vi "PID control for simple Suspension System.vi"() -> ()   [LabVIEW 2014]
uses:
  <vilib>/Simulation/Scripting/Companion Diagram/SimConfigNode/SimParams.ctl
  <vilib>/Simulation/Scripting/Companion Diagram/SimConfigNode/_simSolvers.ctl
  <vilib>/Simulation/Implementation/Shared/SIMSCR Execution Mode.ctl
  <vilib>/Simulation/Param Hierarchy/Typedefs/SIMPH Param Control Actions.ctl
  <vilib>/Simulation/Implementation/Shared/SIM limit type.ctl
  <vilib>/Simulation/Implementation/Shared/NILVSim_ParamChanged.vi
  <vilib>/Simulation/Implementation/Shared/NILVSIM_BeginStep.vi
  <vilib>/Simulation/DataSources/Implementation/NILVSim Step.llb/SIM Step (scalar).vi
  <vilib>/Simulation/ContinuousLinear/Implementation/NILVSim Integrator new.llb/SIM Integrator distributor (scalar).vi
  <vilib>/Simulation/SignalDisplay/Implementation/NILVSim Time Waveform.llb/SIM Time Waveform (vector).vi
  <vilib>/Simulation/Utility/Implementation/NILVSim Memory.llb/NILVSim Memory (core).vi
  <vilib>/Simulation/SignalArithmetic/Implementation/NILVSim Gain.llb/SIM Gain (scalar).vi
  <vilib>/Simulation/ContinuousLinear/Implementation/NILVSim Derivative.llb/SIM derivative (scalar).vi
  <vilib>/Simulation/ContinuousLinear/Implementation/NILVSim Integrator new.llb/SIM Integrator collector (scalar).vi
  <vilib>/Simulation/Implementation/Shared/NILVSim_Manager.vi
  <vilib>/Utility/error.llb/Clear Errors.vi
  <vilib>/Simulation/Implementation/Shared/NILVSim_FinalizeModel.vi
  <vilib>/Simulation/Implementation/Shared/SIM Unbundle Sim Info.vi
  <vilib>/Simulation/Implementation/Shared/NILVSim_Initialize.vi
  <vilib>/Simulation/Utility/Implementation/NILVSim Get Time and IsAcceptedStep.vi
  <vilib>/Simulation/Implementation/Shared/SIMSH Read Queue.vi
  <vilib>/Simulation/Implementation/Shared/NILVSim_GetModelError.vi
  <vilib>/Simulation/Implementation/Shared/SIM Bundle Sim Info.vi
  <vilib>/imath/engines/lvmath/Plug In/Control Design/BuiltInFunctions/tf/NIMS_CD_tf(num,den,Ts).vi
  <vilib>/imath/engines/lvmath/Plug In/Control Design/BuiltInFunctions/plus/NIMS_CD_plus(TF,TF).vi
  <vilib>/imath/engines/lvmath/Functions/Error Handling/MergeErrorsWrapper.vi
  <vilib>/imath/engines/lvmath2/RunTimeEngine/NodeEndStatement/NIMS_NodeEndStatement_Output.vi
  <instcachedir>/0/NIMS_NodeEndStatement_Output_53EC0D466D134D7ABD903AC30B43404B.lvgen/NIMS_NodeEndStatement_Output_53EC0D466D134D7ABD903AC30B43404B_011.vi
  <vilib>/imath/engines/lvmath2/RunTimeEngine/ErrorHandling/NIMS_Finalize Error.vi
  <vilib>/addons/Control Design/_Utility/Model Viewer.llb/Model Viewer SubVI/cd_Draw Transfer Function Equation (TF).vi
  <vilib>/imath/engines/lvmath/Plug In/Control Design/BuiltInFunctions/multmx/NIMS_CD_multmx(TF,TF).vi
  <vilib>/imath/engines/lvmath/Plug In/Control Design/BuiltInFunctions/plus/NIMS_CD_plus(K,TF).vi
  <vilib>/imath/engines/lvmath/Plug In/Control Design/BuiltInFunctions/rightdivmx/NIMS_CD_rightdivmx(TF,TF).vi
  <vilib>/addons/Control Design/_Time Response Analysis/Time Response.llb/Time Response subVI/cd_Step Response (Transfer Function).vi
  <vilib>/Simulation/Scripting/Companion Diagram/SimConfigNode/SimDog.xnode
  <vilib>/Simulation/Implementation/XNodeFramework/SimXNode/SimX.xnode
  <vilib>/Simulation/ContinuousLinear/Implementation/NILVSim Integrator new.llb/SIM Integrator (scalar).vi
  <vilib>/addons/Control Design/_Utility/NI_CD_Model Viewer.lvlib
  <vilib>/addons/Control Design/_Time Response Analysis/NI_CD_Time Response.lvlib
  <vilib>/Simulation/Implementation/Shared/NI_SIM_Implementation.lvlib
panel:
  out "Step Response Graph":cluster{"time":dbl[], dbl[]}[](graph)
  out "Sys Transfer Function":picture
  out "Plant Transfer Function":picture
  out "Waveform Chart":waveform(dbl)[](graph)=[{"t0"=timestamp(15 s since 1904-01-01), "dt"=1.0, "Y"=[1.0]}, {"t0"=timestamp(15 s since 1904-01-01), "dt"=1.0, "Y"=[1.0087547383688724]}, {"t0"=timestamp(15 s since 1904-01-01), "dt"=1.0, "Y"=[0.0038100438574991146]}]
  in  "Control Parameters":cluster{"Kp":dbl, "TI":dbl, "TD":dbl}={"Kp"=12.0, "TI"=5.0, "TD"=1.0}
  out "PID Transfer Function":picture
  in  "System Parameters":T1={"m[kg]"=10.0, "k[N/m]"=0.01, "d[N*s/m]"=10.0}
  # "Title: PID control loop, Bond Graph\nAuthor: Jad Saud FOXYVM \nDate: 2019.11.19\nVersion: v1.0"
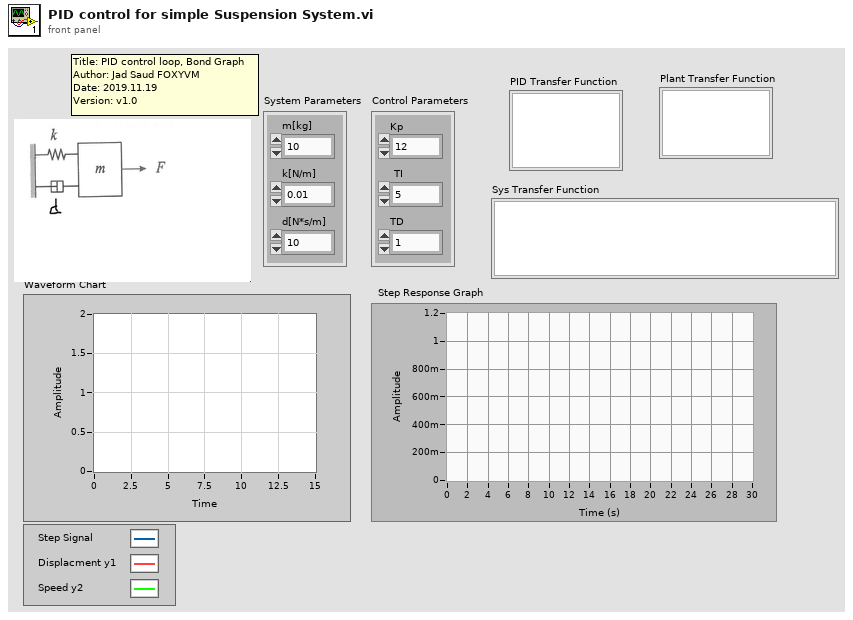
[diagram p1: front panel]
types:
  T1 = cluster{"m[kg]":dbl, "k[N/m]":dbl, "d[N*s/m]":dbl}
  T2 = typedef "NI_LinSys_Model Typedefs.lvlib/CD Transfer Function Model (MIMO).ctl" = cluster{"properties":T3, "transfer function(s)":T4[][]}
  T3 = typedef "NI_LinSys_Model Typedefs.lvlib/CD General Elements.ctl" = cluster{"Model name":string, "Input names":string[], "Output names":string[], "Input Delays":dbl[], "Output Delays":dbl[], "Sampling Time":dbl, "Notes":string}
  T4 = typedef "NI_LinSys_Model Typedefs.lvlib/CD Transfer Function Model (SISO).ctl" = cluster{"Numerator":dbl[], "Denominator":dbl[], "delay":dbl}
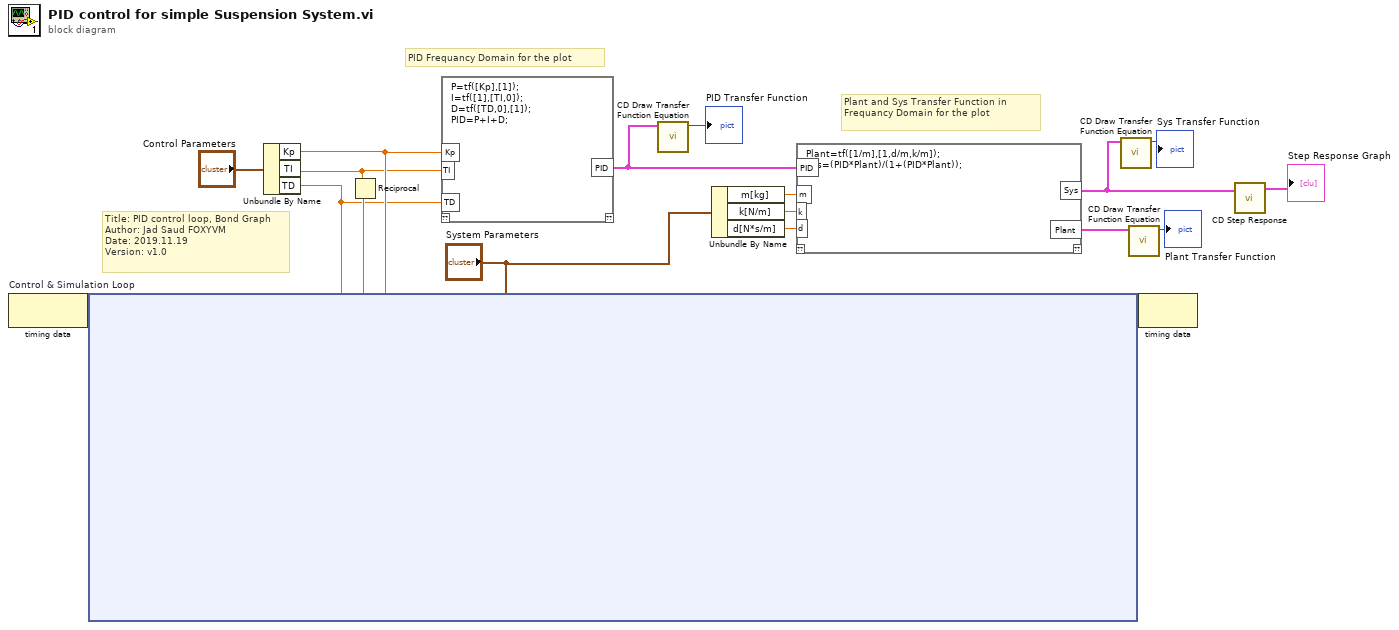
[diagram p0: block diagram]
diagram:
  # "Plant and Sys Transfer Function in Frequancy Domain for the plot"
  # "Title: PID control loop, Bond Graph\nAuthor: Jad Saud FOXYVM \nDate: 2019.11.19\nVersion: v1.0"
  # "PID Frequancy Domain for the plot"
  n1 = node-c288() -> (w18:variant)  [unwired: 1 in]
  n2 = Unbundle By Name ("Unbundle By Name 2")("Control Parameters") -> ("Kp"=w13:dbl, "TI"=w12:dbl, "TD"=w11:dbl)
  n3 = Reciprocal(x=w12) -> (1/x=w16:dbl)
  n4 = node-c254 "Control & Simulation Loop"(w18, w16, "System Parameters", w13, w11) -> (w17:variant)
  n5 = mathscript code="P=tf([Kp],[1]);\nI=tf([1],[TI,0]);\nD=tf([TD,0],[1]);\nPID=P+I+D;"("Kp"=w13, "TI"=w12, "TD"=w11) -> ("PID"=w10:T2)  [unwired: 1 in, 1 out]
  n6 = call-poly <vilib>:"CD Draw Transfer Function Equation.vi"("Transfer Function Model"=w10) -> ("Equation"=→"PID Transfer Function":picture)  [unwired: 8 in, 2 out]
  n7 = Unbundle By Name ("Unbundle By Name 2")("System Parameters") -> ("m[kg]"=w6:dbl, "k[N/m]"=w5:dbl, "d[N*s/m]"=w4:dbl)
  n8 = mathscript code="Plant=tf([1/m],[1,d/m,k/m]);\nSys=(PID*Plant)/(1+(PID*Plant));"("m"=w6, "k"=w5, "d"=w4, "PID"=w10) -> ("Plant"=w8:T2, "Sys"=w2:T2)  [unwired: 1 in, 1 out]
  n9 = call-poly <vilib>:"CD Draw Transfer Function Equation.vi"("Transfer Function Model"=w2) -> ("Equation"=→"Sys Transfer Function":picture)  [unwired: 8 in, 2 out]
  n10 = call-poly <vilib>:"CD Draw Transfer Function Equation.vi"("Transfer Function Model"=w8) -> ("Equation"=→"Plant Transfer Function":picture)  [unwired: 8 in, 2 out]
  n11 = node-c288(w17) -> ()  [unwired: 1 out]
  n12 = call-poly <vilib>:"CD Step Response.vi"("Transfer Function Model"=w2) -> ("Step Response Graph"=→"Step Response Graph":cluster{"time":dbl[], dbl[]}[])  [unwired: 8 in, 2 out]
